vi "Get Library in Project.vi"(7 "Error if Not Found? (F)":bool=TRUE, 8 "error in (no error)":errorcluster, 10 "Measurement Service Name":string, 11 "Project in":refnum<vi>) -> (0 "error out":errorcluster, 1 "Found?":bool, 2 "Measurement Library Item":refnum<vi>)   [LabVIEW 2020]
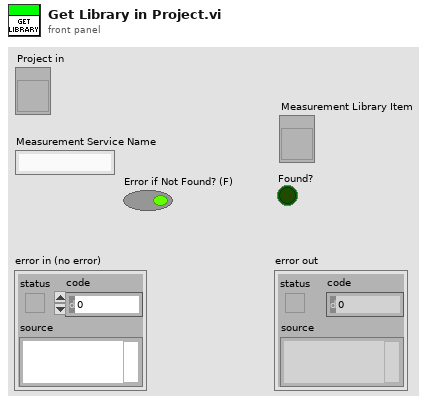
[diagram p1: front panel]
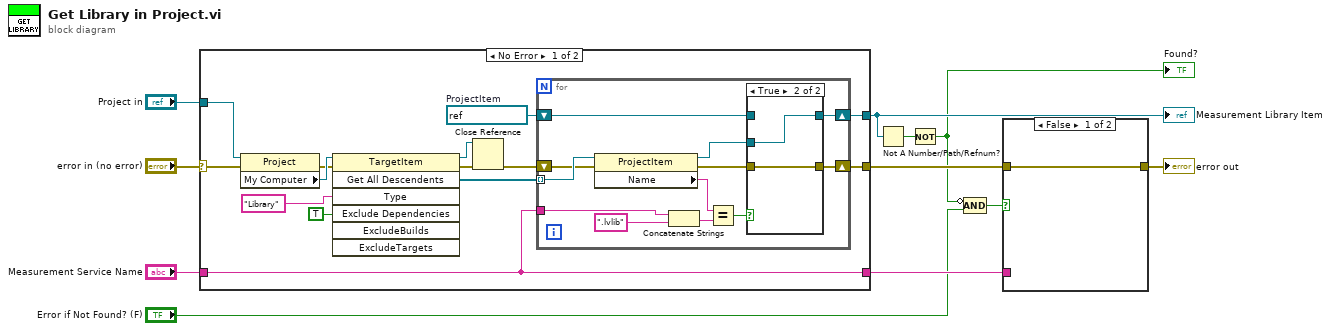
[diagram p0: block diagram]
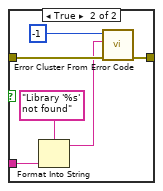
[diagram p2: hidden frame]
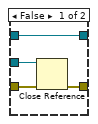
[diagram p3: hidden frame]
diagram:
  n1 = case shown="No Error" "error in (no error)" {
    selector: "error in (no error)" -> [w21 w45]
    tunnel: "Project in" -> [w25 _]
    tunnel: "Measurement Service Name" -> [w13 w44]
    tunnel: [w20 w45] -> w6
    tunnel: [w15 _] -> w8
    tunnel: [w13 w44] -> w5
    frame No Error {
      w16 = refnum<vi> refnum  # ProjectItem
      n2 = property class="Project"(reference=w25, error in=w21) -> (error out=w23:errorcluster, "My Computer"=w24:refnum<vi>)  [unwired: 1 out]
      n3 = invoke class="TargetItem" method="Get All Descendents"(reference=w24, error in=w23, "Type"="Library", "Exclude Dependencies"=TRUE ("ExcludeDependencies")) -> (reference out=w18:refnum<vi>, error out=w19:errorcluster, "All Descendents"=w22:refnum<vi>[])  [unwired: 3 in, 4 out]
      n4 = Close Reference(reference=w18, error in (no error)=w19) -> (error out=w17:errorcluster)
      n5 = for {
        tunnel: w22 -> [w37] mode=indexing
        tunnel: w13 -> [w36]
        shift-right: [w28] -> w20
        shift-left: w17 -> [w32]
        shift-right: [w27] -> w15
        shift-left: w16 -> [w26]
        n6 = property class="ProjectItem"(reference=w37, error in=w32) -> (reference out=w30:refnum<vi>, error out=w31:errorcluster, "Name"=w34:string)
        n7 = Concatenate Strings(w36, ".lvlib" ("string")) -> (w33:string)
        n8 = Equal?(x=w34, y=w33) -> (x = y?=w29:bool)
        n9 = case shown="True" w29 {
          tunnel: w31 -> [w41 w43]
          tunnel: w30 -> [w38 w42]
          tunnel: [w40 w43] -> w28
          tunnel: [w39 w42] -> w27
          tunnel: w26 -> [w39 _]
          frame False {
            n10 = Close Reference(reference=w38, error in (no error)=w41) -> (error out=w40:errorcluster)
          }
          frame True {
          }
        }
      }
    }
    frame Error {
    }
  }
  "Measurement Library Item" <- w8
  n11 = Not A Number/Path/Refnum?(number/path/refnum=w8) -> (NaN/Path/Refnum?=w4:bool)
  n12 = Not(x=w4) -> (.not. x?=w2:bool)
  "Found?" <- w2
  n13 = Compound Arithmetic op=AND(invert w2, "Error if Not Found? (F)") -> (w3:bool)
  n14 = case shown="False" w3 {
    tunnel: [w46 w52] -> w7
    tunnel: w6 -> [w46 w51]
    tunnel: w5 -> [_ w47]
    frame False {
    }
    frame True {
      n15 = Format Into String(format string="Library '%s' not found" ("initial string"), w47) -> (resulting string=w48:string)  [unwired: 2 in, 1 out]
      n16 = call <vilib>:"Error Cluster From Error Code.vi"("error in (no error)"=w51, "error message (\"\")"=w48, "error code (0)"=-1) -> ("error out"=w52:errorcluster)  [unwired: 6 in]
    }
  }
  "error out" <- w7
